vi "Set Settings.vi"(8 "error in (no error)":errorcluster, 10 "Settings":T1, 11 "Database in":refnum<class "Database.lvclass">) -> (0 "error out":errorcluster, 3 "Database out":refnum<class "Database.lvclass">)   [LabVIEW 2022 SP3, in "Database.lvclass"]
doc: "Developed by Kevin Thompson\nkevin@thompsonengineering.net\n\nCopyright 2018\nThompson Engineering, LLC"
uses:
  Database.lvclass
  DataTypes/Settings--cluster.ctl
  Database.lvclass/Database.ctl
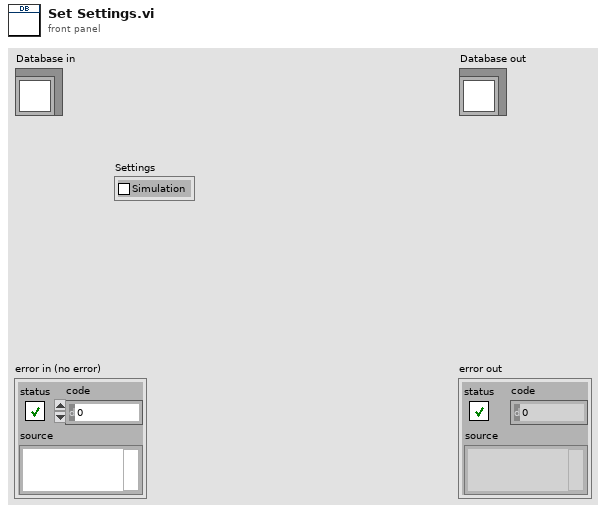
[diagram p1: front panel]
types:
  T1 = typedef "Database.lvclass/Settings--cluster.ctl" = cluster{"Simulation":bool}
  T2 = typedef "Database.lvclass/ObjData--cluster.ctl" = cluster{"Settings":T1, "Public Events":T3, "Dependency":T4, "ReadData-placeholder":T5, "VISA-placeholder":refnum<visa-resource-name>}
  T3 = typedef "Database.lvclass/Public Events--cluster.ctl" = cluster{"Temp01.AsyncCmd Event":refnum<user-event>, "Temp01.AsyncMsg Event":refnum<user-event>, "stop process":refnum<user-event>, "API Incoming Event":refnum<user-event>, "API Executed Event":refnum<user-event>, "API Return Event":refnum<user-event>}
  T4 = typedef "Database.lvclass/Dependency--cluster.ctl" = cluster{"Config":refnum<class>, "ClassRef":refnum<class>}
  T5 = typedef "Database.lvclass/Read Data--cluster.ctl" = cluster{"Data":dbl}
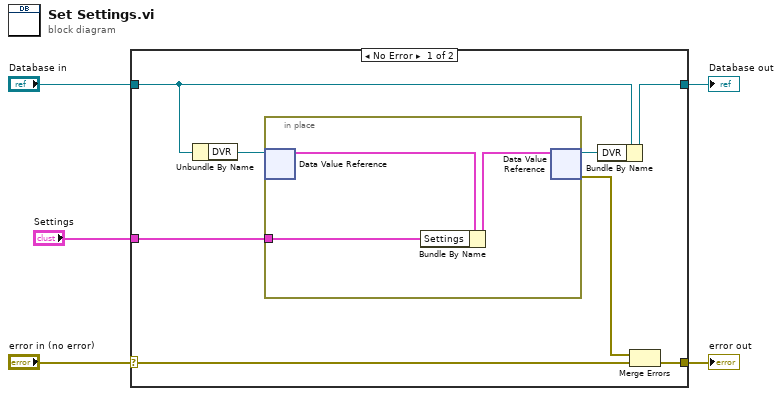
[diagram p0: block diagram]
diagram:
  n1 = case shown="No Error" "error in (no error)" {
    selector: "error in (no error)" -> [w13 w17]
    tunnel: [w8 w17] -> w4
    tunnel: [w9 w18] -> w2
    tunnel: "Database in" -> [w12 w18]
    tunnel: "Settings" -> [w6 _]
    frame No Error {
      n2 = Unbundle By Name(w12) -> ("DVR"=w11:refnum<data-value>)
      n3 = in-place {
        in-place-border: w6 -> [w14]
        n4 = in-place-dvr #1(w11) -> (w16:T2)  [unwired: 1 out]
        n5 = Bundle By Name(cluster=w16, "Settings"=w14) -> (w15:T2)
        n6 = in-place-dvr #1(w15) -> (w10:refnum<data-value>, w7:errorcluster)
      }
      n7 = Bundle By Name(cluster=w12, "DVR"=w10) -> (w9:refnum<class "Database.lvclass">)
      n8 = Merge Errors(w7, w13) -> (w8:errorcluster)
    }
    frame Error {
    }
  }
  "error out" <- w4
  "Database out" <- w2
